vi "Remove Channel.vi"(7 "Type":T1, 8 "error in (no error)":errorcluster, 10 "Channel Name":string, 11 "User BluelinesRedlines in":refnum<class "User BluelinesRedlines.lvclass">) -> (0 "error out":errorcluster, 3 "User BluelinesRedlines out":refnum<class "User BluelinesRedlines.lvclass">)   [LabVIEW 2020, in "VolatusGUIElements.lvlib" / "User BluelinesRedlines.lvclass"]
uses:
  User BluelinesRedlines.lvclass
  User BluelinesRedlines.lvclass/User BluelinesRedlines.ctl
  VolatusGUI/BluelinesRedlines Source/BLRL Type.ctl
  VolatusGUI/BluelinesRedlines Source/BluelinesRedlines Source.lvclass
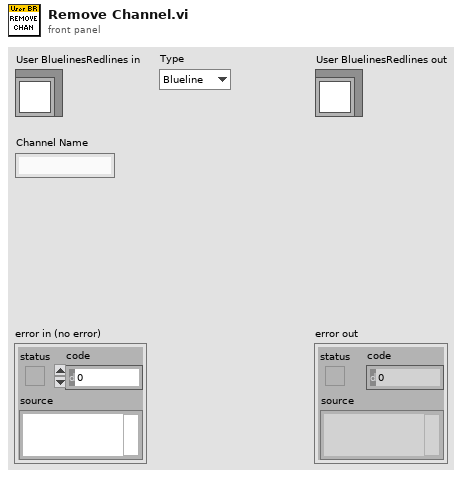
[diagram p1: front panel]
types:
  T1 = typedef "VolatusGUI.lvlib/BluelinesRedlines Source.lvclass/BLRL Type.ctl" = enum16{"Blueline", "Redline"}
  T2 = typedef "VolatusGUI.lvlib/BluelinesRedlines Source.lvclass/Range Limit Config.ctl" = cluster{"Channel":string, "Low Limit":dbl, "High Limit":dbl}
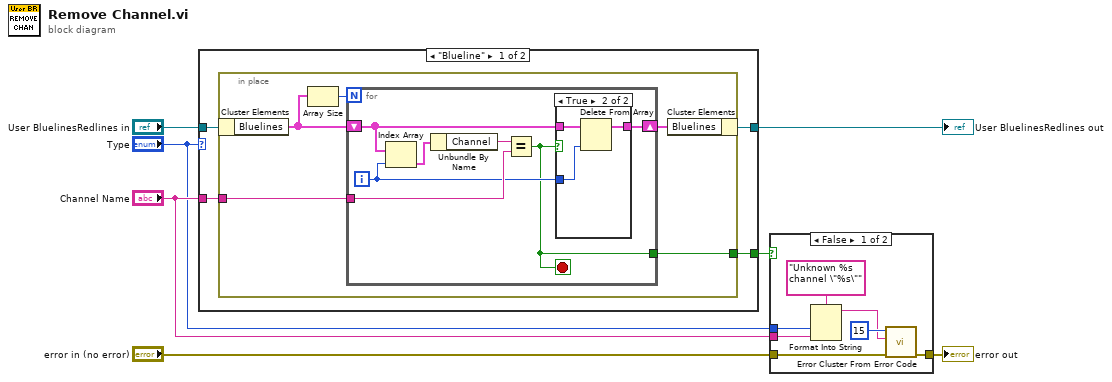
[diagram p0: block diagram]
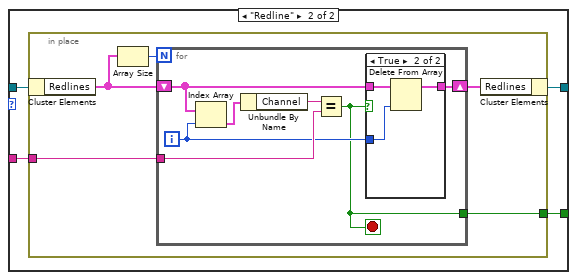
[diagram p3: hidden frame]
diagram:
  n1 = case shown="\"Blueline\"" "Type" {
    tunnel: "User BluelinesRedlines in" -> [w11 w31]
    tunnel: [w10 w30] -> w6
    tunnel: "Channel Name" -> [w9 w29]
    tunnel: [w8 w28] -> w5
    frame "Blueline" {
      n2 = in-place {
        in-place-border: w9 -> [w13]
        in-place-border: [w12] -> w8
        n3 = in-place-cluster #1(w11) -> ("Bluelines"=w14:T2[])
        n4 = Array Size(array=w14) -> (size(s)=w15:i32)
        n5 = for {
          N: w15 -> [_]
          shift-right: [w18] -> w16
          shift-left: w14 -> [w21]
          tunnel: w13 -> [w22]
          tunnel: [w17] -> w12
          i -> [w20]
          stop <- w17 stop-if-true
          n6 = Index Array(array=w21, index=w20) -> (element=w19:T2)
          n7 = Unbundle By Name(w19) -> ("Channel"=w23:string)
          n8 = Equal?(x=w23, y=w22) -> (x = y?=w17:bool)
          n9 = case shown="True" w17 {
            tunnel: w21 -> [w24 w27]
            tunnel: w20 -> [_ w25]
            tunnel: [w24 w26] -> w18
            frame False {
            }
            frame True {
              n10 = Delete From Array(array=w27, index=w25) -> (array with subset deleted=w26:T2[])  [unwired: 1 in, 1 out]
            }
          }
        }
        n11 = in-place-cluster #1("Bluelines"=w16) -> (w10:refnum<class "User BluelinesRedlines.lvclass">)
      }
    }
    frame "Redline" {
      n12 = in-place {
        in-place-border: w29 -> [w33]
        in-place-border: [w32] -> w28
        n13 = in-place-cluster #2(w31) -> ("Redlines"=w34:T2[])
        n14 = Array Size(array=w34) -> (size(s)=w35:i32)
        n15 = for {
          N: w35 -> [_]
          shift-right: [w38] -> w36
          shift-left: w34 -> [w41]
          tunnel: w33 -> [w42]
          tunnel: [w37] -> w32
          i -> [w40]
          stop <- w37 stop-if-true
          n16 = Index Array(array=w41, index=w40) -> (element=w39:T2)
          n17 = Unbundle By Name(w39) -> ("Channel"=w43:string)
          n18 = Equal?(x=w43, y=w42) -> (x = y?=w37:bool)
          n19 = case shown="True" w37 {
            tunnel: w41 -> [w44 w47]
            tunnel: w40 -> [_ w45]
            tunnel: [w44 w46] -> w38
            frame False {
            }
            frame True {
              n20 = Delete From Array(array=w47, index=w45) -> (array with subset deleted=w46:T2[])  [unwired: 1 in, 1 out]
            }
          }
        }
        n21 = in-place-cluster #2("Redlines"=w36) -> (w30:refnum<class "User BluelinesRedlines.lvclass">)
      }
    }
  }
  "User BluelinesRedlines out" <- w6
  n22 = case shown="False" w5 {
    tunnel: "error in (no error)" -> [w51 w55]
    tunnel: "Channel Name" -> [w54 _]
    tunnel: "Type" -> [w53 _]
    tunnel: [w48 w55] -> w1
    frame False {
      n23 = Format Into String(format string="Unknown %s channel \"%s\"", w53, w54) -> (resulting string=w49:string)  [unwired: 2 in, 1 out]
      n24 = call <vilib>:"Error Cluster From Error Code.vi"("error in (no error)"=w51, "error message (\"\")"=w49, "error code (0)"=15) -> ("error out"=w48:errorcluster)  [unwired: 6 in]
    }
    frame True {
    }
  }
  "error out" <- w1
